vi "CAL_SET_SHOT_AUTON_1.vi"(7 "arguments":string[](array[string]), 8 "dt":i32, 9 "Reinit":bool, 10 "bus_inputs":T1={"dt_enc_left_dist"=0.0, "dt_enc_right_dist"=0.0, "dt_enc_left_spd"=0.0, "dt_enc_right_spd"=0.0, "veh_spd"=0.0, "dt_gyro_hdg"=0.0, "dt_gyro_spd"=0.0, "coll_choo_choo_pos"=0.0, "rbt_press_sw"=FALSE, "rbt_batt_vsup"=0.0, "rbt_ana_vref"=1.0, "rbt_dig_vsup"=0.0, "coll_spring_adj_pos"=0.0, "coll_ball_sw"=FALSE, "coll_up_sw"=FALSE}, 11 "bus_state":T2) -> (1 "Done":bool, 2 "bus_inputs out":T1={"dt_enc_left_dist"=0.0, "dt_enc_right_dist"=0.0, "dt_enc_left_spd"=0.0, "dt_enc_right_spd"=0.0, "veh_spd"=0.0, "dt_gyro_hdg"=0.0, "dt_gyro_spd"=0.0, "coll_choo_choo_pos"=0.0, "rbt_press_sw"=FALSE, "rbt_batt_vsup"=0.0, "rbt_ana_vref"=1.0, "rbt_dig_vsup"=0.0, "coll_spring_adj_pos"=0.0, "coll_ball_sw"=FALSE, "coll_up_sw"=FALSE}, 3 "bus_state out":T2)   [LabVIEW 2013]
uses:
  structures/bus_state.ctl
  structures/bus_state_drivetrain.ctl
  structures/bus_state_collector.ctl
  collector/collector_shot_cal.ctl
  structures/bus_inputs.ctl
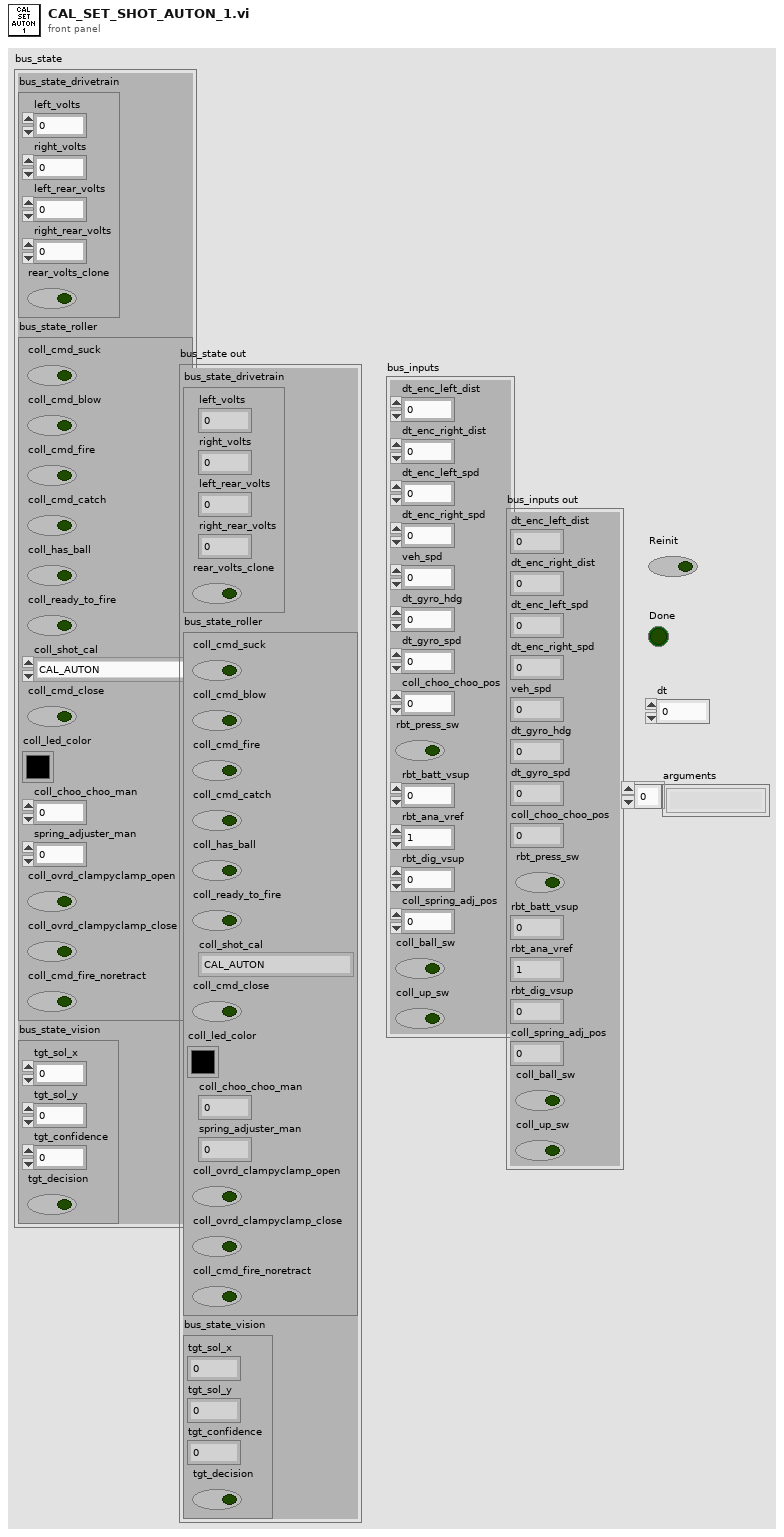
[diagram p1: front panel]
types:
  T1 = typedef "bus_inputs.ctl" = cluster{"dt_enc_left_dist":sgl, "dt_enc_right_dist":sgl, "dt_enc_left_spd":sgl, "dt_enc_right_spd":sgl, "veh_spd":sgl, "dt_gyro_hdg":sgl, "dt_gyro_spd":sgl, "coll_choo_choo_pos":sgl, "rbt_press_sw":bool, "rbt_batt_vsup":sgl, "rbt_ana_vref":dbl, "rbt_dig_vsup":dbl, "coll_spring_adj_pos":sgl, "coll_ball_sw":bool, "coll_up_sw":bool}
  T2 = typedef "bus_state.ctl" = cluster{"bus_state_drivetrain":T3, "bus_state_roller":T4, "bus_state_vision":cluster{"tgt_sol_x":dbl, "tgt_sol_y":dbl, "tgt_confidence":dbl, "tgt_decision":bool}}
  T3 = typedef "bus_state_drivetrain.ctl" = cluster{"left_volts":sgl, "right_volts":sgl, "left_rear_volts":sgl, "right_rear_volts":sgl, "rear_volts_clone":bool}
  T4 = typedef "bus_state_collector.ctl" = cluster{"coll_cmd_suck":bool, "coll_cmd_blow":bool, "coll_cmd_fire":bool, "coll_cmd_catch":bool, "coll_has_ball":bool, "coll_ready_to_fire":bool, "coll_shot_cal":T5, "coll_cmd_close":bool, "coll_led_color":u32, "coll_choo_choo_man":sgl, "spring_adjuster_man":sgl, "coll_ovrd_clampyclamp_open":bool, "coll_ovrd_clampyclamp_close":bool, "coll_cmd_fire_noretract":bool}
  T5 = typedef "collector_shot_cal.ctl" = enum16{"CAL_AUTON", "CAL_CLOSE", "CAL_MID", "CAL_FAR", "NOT_SAFE_TO_ACTUATE"}
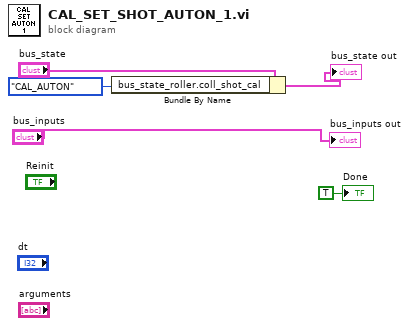
[diagram p0: block diagram]
diagram:
  n1 = Bundle By Name(cluster="bus_state", "bus_state_roller.coll_shot_cal"=collector_shot_cal."CAL_AUTON") -> (→"bus_state out":T2)
  "bus_inputs out" <- "bus_inputs"
  "Done" <- TRUE ("Done")
